vi "GetStatus.vi"(8 "error in (no error)":errorcluster, 11 "Value":string) -> (0 "error out":errorcluster, 2 "status":string, 3 "Found":bool)   [LabVIEW 2021]
uses:
  b3b0fdf2-cb34-410b-9075-fd36f45b70f0.vi
  <vilib>/JDP Science/JSONtext/Find Item.vi
  <vilib>/JDP Science/JSONtext/Next JSON Value.vi
  <vilib>/JDP Science/JSONtext/String Subset.vi
  <vilib>/JDP Science/JSONtext/Parsing/Advance past next JSON Value (inlined COPY).vi
  <vilib>/JDP Science/JSONtext/Parsing/Advance past whitespace.vi
  <vilib>/JDP Science/JSONtext/Parsing/Advance past String.vi
  <vilib>/JDP Science/JSONtext/Parsing/Advance past Number.vi
  <vilib>/JDP Science/JSONtext/Parsing/Advance past Line Ending.vi
  <vilib>/JDP Science/JSONtext/Parsing/Parse Full Path or Item Name.vi
  <vilib>/JDP Science/JSONtext/Parsing/Advance past Array.vi
  <vilib>/JDP Science/JSONtext/Parsing/Advance past Object.vi
  <vilib>/JDP Science/JSONtext/support/Error Cluster From Code.vi
  <vilib>/JDP Science/JSONtext/Offset/Find Item Locations by Path.vi
  <vilib>/JDP Science/JSONtext/JSON text to Variant.vi
  <vilib>/JDP Science/JSONtext/LVClass Serializer/JSONtext LVClass Serializer.lvclass
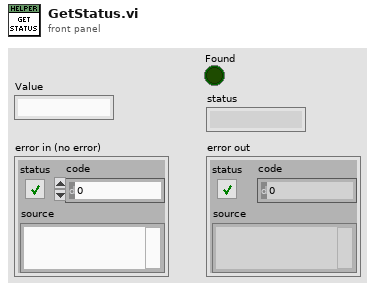
[diagram p1: front panel]
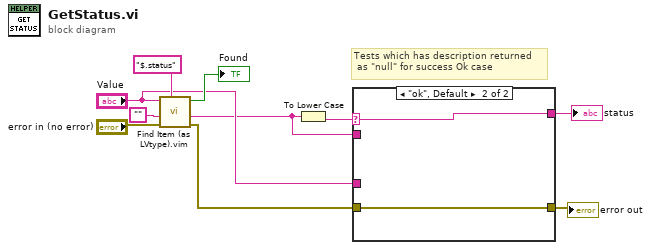
[diagram p0: block diagram]
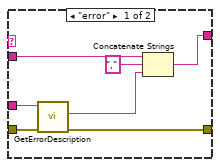
[diagram p2: hidden frame]
diagram:
  # "Tests which has description returned\n as \"null\" for success Ok case"
  n1 = call "Find Item (as LVtype).vim"("$Path or Item Name"="$.status", "error in (no error)"="error in (no error)", "Data Type and Default Value"="", "JSON"="Value") -> ("error out"=w5:errorcluster, "Data"=w1:string, "Found"=→"Found":bool)  [unwired: 4 in, 1 out]
  n2 = To Lower Case(string=w1) -> (all lower case string=w6:string)
  n3 = case shown="\"ok\", Default" w6 {
    selector: w6 -> [_ w19]
    tunnel: [w17 w18] -> w3
    tunnel: [w11 w19] -> w2
    tunnel: w5 -> [w16 w18]
    tunnel: "Value" -> [w15 _]
    tunnel: w1 -> [w14 _]
    frame "error" {
      n4 = call "GetErrorDescription.vi"("error in (no error)"=w16, "Value"=w15) -> ("error out"=w17:errorcluster, "description"=w12:string)  [unwired: 7 in, 1 out]
      n5 = Concatenate Strings(w14, "," ("string"), w12) -> (w11:string)
    }
    frame "ok", Default {
    }
  }
  "error out" <- w3
  "status" <- w2
